vi "logService.vi"() -> ()   [LabVIEW 2014]
uses:
  R/manifest.vi
panel:
  out "error IO":errorcluster
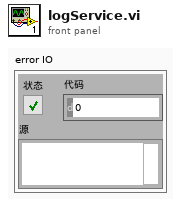
[diagram p1: front panel]
types:
  T1 = cluster{"标题":string, "相对路径":string, "类型":enum16{"服务", "活动"}, "专属队列名称":string}
  T2 = enum16{"open", "replace", "create", "open or create", "replace or create", "replace or create with confirmation"}
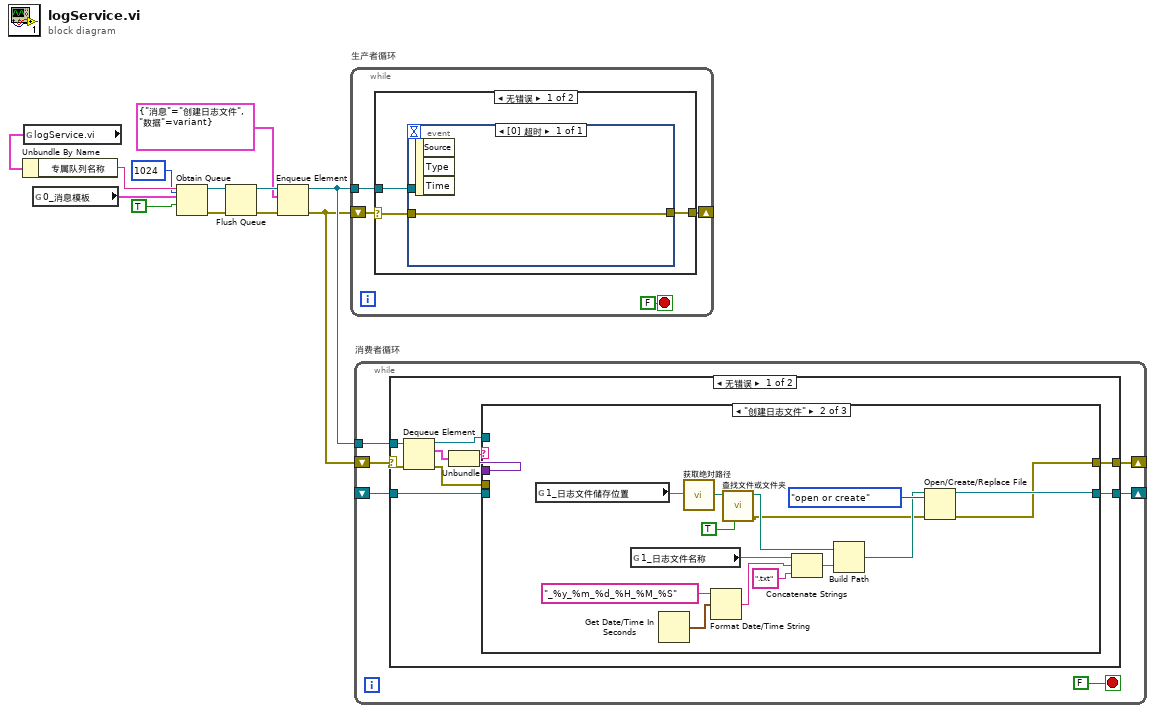
[diagram p0: block diagram]
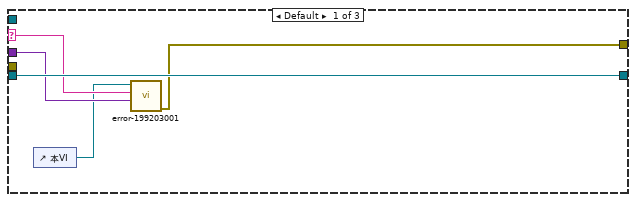
[diagram p2: hidden frame]
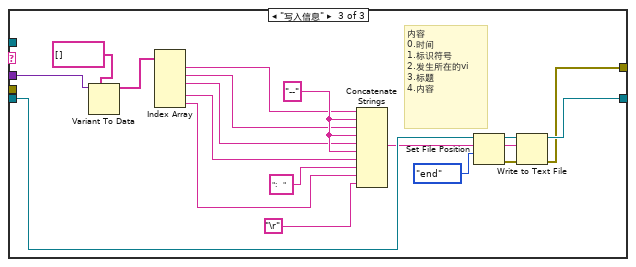
[diagram p3: hidden frame]
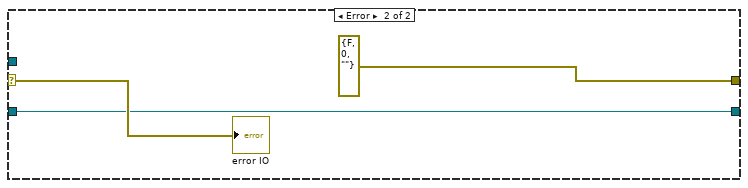
[diagram p4: hidden frame]
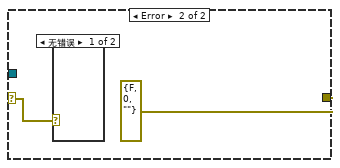
[diagram p5: hidden frame]
diagram:
  n1 = global read "manifest.vi" "logService.vi"() -> (w12:T1)
  n2 = Unbundle By Name(w12) -> ("专属队列名称"=w11:string)
  n3 = global read "manifest.vi" "0_消息模板"() -> (w10:cluster{"消息":string, "数据":variant})
  n4 = Obtain Queue(max queue size (-1, unlimited)=1024 ("队列最大值（-1，无限）"), name (unnamed)=w11, element data type=w10, create if not found? (T)=TRUE ("如未找到是否创建？(T)")) -> (queue out=w6:refnum<queue>, error out=w7:errorcluster)  [unwired: 1 in, 1 out]
  n5 = Flush Queue(queue=w6, error in (no error)=w7) -> (queue out=w4:refnum<queue>, error out=w5:errorcluster)  [unwired: 1 out]
  n6 = Enqueue Element(queue=w4, element=cluster{"消息":string, "数据":variant} {"消息"="创建日志文件", "数据"=variant} ("元素"), error in (no error)=w5) -> (queue out=w2:refnum<queue>, error out=w1:errorcluster)  [unwired: 1 in, 1 out]
  n7 = while "生产者循环" {
    tunnel: w2 -> [w15]
    shift-right: [w14] -> _
    shift-left: w1 -> [w16]
    stop <- FALSE stop-if-true
    n8 = case shown="无错误" w16 {
      selector: w16 -> [w18 w21]
      tunnel: w15 -> [w19 _]
      tunnel: [w17 errorcluster {"status"=FALSE, "code"=0, "source"=""} ("错误常量")] -> w14
      frame No Error {
        n9 = event shown="[0] 超时" {
          selector: _ -> [_]
          dyn-events: _ -> [_]
          timeout: _ -> [_]
          tunnel: w19 -> [_]
          tunnel: w18 -> [w20]
          tunnel: [w20] -> w17
          event Timeout {
            n10 = event-data() -> ()  [unwired: 1 in, 3 out]
          }
        }
      }
      frame Error {
        n11 = case shown="无错误" w21 {
          frame No Error {
          }
          frame Error {
          }
        }
      }
    }
  }
  n12 = while "消费者循环" {
    tunnel: w2 -> [w27]
    shift-right: [w26] -> _
    shift-left: w1 -> [w28]
    shift-right: [w24] -> _
    shift-left: _ -> [w23]
    stop <- FALSE stop-if-true
    n13 = case shown="无错误" w28 {
      selector: w28 -> [w38 w78]
      tunnel: w27 -> [w37 _]
      tunnel: [w31 errorcluster {"status"=FALSE, "code"=0, "source"=""} ("1992021")] -> w26
      tunnel: [w30 w77] -> w24
      tunnel: w23 -> [w29 w77]
      frame No Error {
        n14 = Dequeue Element(queue=w37, error in (no error)=w38) -> (queue out=w32:refnum<queue>, element=w36:cluster{"消息":string, "数据":variant}, error out=w33:errorcluster)  [unwired: 1 in, 1 out]
        n15 = Unbundle(w36) -> ("消息"=w35:string, "数据"=w34:variant)
        n16 = case shown="\"创建日志文件\"" w35 {
          selector: w35 -> [w42 _ _]
          tunnel: w34 -> [w41 _ w75]
          tunnel: w33 -> [_ _ _]
          tunnel: w32 -> [_ _ _]
          tunnel: [w40 w50 w59] -> w31
          tunnel: [w43 w51 w66] -> w30
          tunnel: w29 -> [w43 _ w71]
          frame Default {
            n17 = control-ref of="本VI"() -> (w39:refnum<vi>)
            n18 = call "error-199203001.vi"("数据"=w41, "字符串"=w42, "VI输入"=w39) -> ("错误输出"=w40:errorcluster)  [unwired: 8 in]
          }
          frame "创建日志文件" {
            n19 = global read "manifest.vi" "1_日志文件储存位置"() -> (w48:string)
            n20 = global read "manifest.vi" "1_日志文件名称"() -> (w49:string)
            n21 = Get Date/Time In Seconds() -> (seconds since 1Jan1904=w58:timestamp)
            n22 = call "获取绝对路径.vi"("relativePath"=w48) -> ("absolutePath"=w47:path)
            n23 = Format Date/Time String(time format string (%c)="_%y_%m_%d_%H_%M_%S" ("时间格式字符串(%c)"), seconds (now)=w58) -> (date/time string=w56:string)  [unwired: 1 in]
            n24 = call "查找文件或文件夹.vi"("create file or folder？"=TRUE, "pathIn"=w47) -> ("error out"=w44:errorcluster, "pathOut"=w45:path)  [unwired: 7 in, 1 out]
            n25 = Concatenate Strings(w49, w56, ".txt" ("字符串")) -> (w54:string)
            n26 = Build Path(base path=w45, name or relative path=w54) -> (appended path=w52:path)
            n27 = Open/Create/Replace File(file path (use dialog)=w52, error in=w44, operation (0:open)=T2."open or create" ("操作(0:open)")) -> (refnum out=w51:refnum<file>, error out=w50:errorcluster)  [unwired: 3 in, 1 out]
          }
          frame "写入信息" {
            w68 = "--" ("字符串")
            # "内容\n0.时间\n1.标识符号\n2.发生所在的vi\n3.标题\n4.内容"
            n28 = Variant To Data(type=string[] [], Variant=w75) -> (data=w67:string[])  [unwired: 1 in, 1 out]
            n29 = Index Array(array=w67) -> (element #1=w64:string, element #2=w63:string, element #3=w62:string, element #4=w61:string, element #5=w60:string)  [unwired: 5 in]
            n30 = Concatenate Strings(w64, w68, w63, w68, w62, w68, w61, ":   " ("字符串"), w60, "\r") -> (w65:string)
            n31 = Set File Position(refnum=w71, from (0:start)=enum16{"start", "end", "current"}."end" ("自（0:起始）")) -> (refnum out=w73:refnum<file>, error out=w74:errorcluster)  [unwired: 2 in]
            n32 = Write to Text File(file (use dialog)=w73, text=w65, error in=w74) -> (refnum out=w66:refnum<file>, error out=w59:errorcluster)  [unwired: 1 in, 1 out]
          }
        }
      }
      frame Error {
        "error IO" <- w78
      }
    }
  }
